vi "test Acyclic Loopback Value Overflow.vi"(8 "error in":errorcluster, 11 "TestCase in":refnum<class "Single Board Loopback.lvclass">) -> (0 "error out":errorcluster, 3 "TestCase out":refnum<class "Single Board Loopback.lvclass">)   [LabVIEW 2020, in "Single Board Loopback.lvclass"]
uses:
  Single Board Loopback.lvclass
  <vilib>/addons/_JKI Toolkits/VI Tester/TestCase.llb/TestCase.lvclass
  <vilib>/NI VeriStand/Execution/Workspace/NI_VS Workspace ExecutionAPI.lvlib
  niveristand-custom-device-testing-tools/VeriStandTestUtilities/VeriStandTestUtilities.lvlib
  <vilib>/NI VeriStand/Execution/Workspace/NI VeriStand - Set Multiple Channel Values.vi
  <vilib>/numeric/Random Number (Range) U64.vi
  C:/Users/nitest/Desktop/Git 2020/niveristand-custom-device-testing-tools/VeriStandTestCase/VeriStandTestCase.lvclass
  C:/Program Files (x86)/National Instruments/LabVIEW 2020/vi.lib/addons/_JKI Toolkits/VI Tester/TestCase.llb/TestCase.lvclass
  C:/Users/nitest/Desktop/Git 2020/niveristand-ballard-arinc429-custom-device/Source/Custom Device Support/Tests/System/Single Board Loopback/Single Board Loopback.lvclass
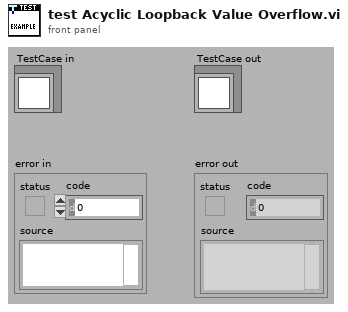
[diagram p1: front panel]
types:
  T1 = typedef "NI_VS Workspace ExecutionAPI.lvlib/WorkspaceAPI.ctl" = refnum<k24>
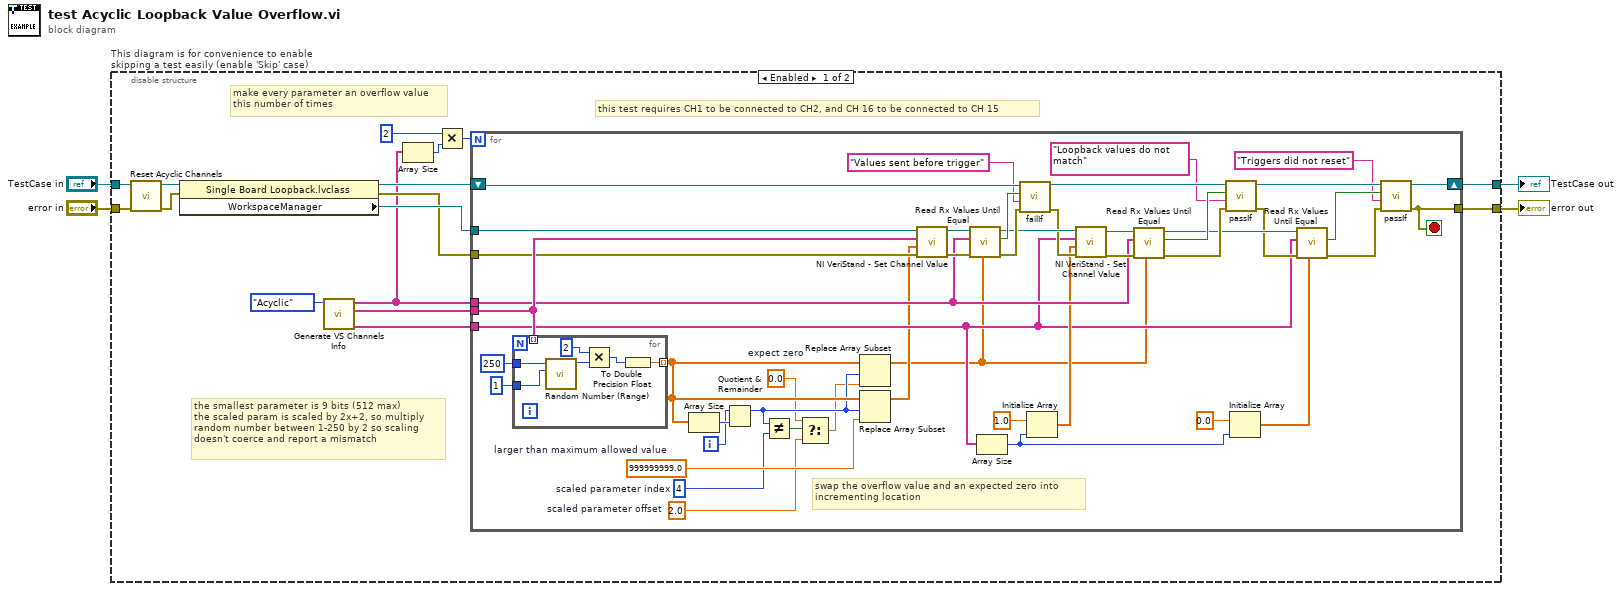
[diagram p0: block diagram]
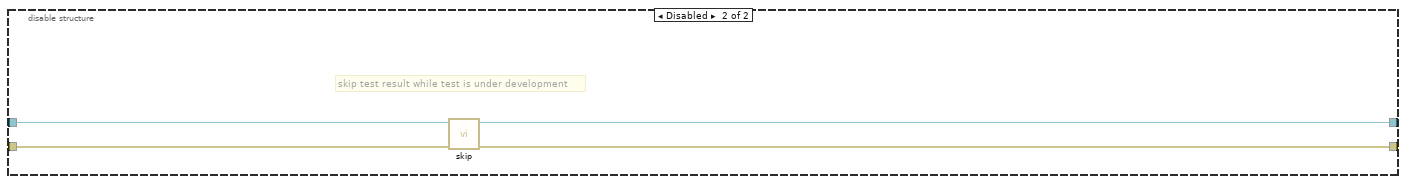
[diagram p2: hidden frame]
diagram:
  n1 = disable-structure "This diagram is for convenience to enable skipping a test easily (enable 'Skip' case)" shown="Enabled" {
    disable-tunnel: "TestCase in" -> [w5 w76]
    disable-tunnel: [w16 w74] -> w1
    disable-tunnel: [w15 w75] -> w3
    disable-tunnel: "error in" -> [w17 w73]
    frame Enabled {
      # "make every parameter an overflow value\nthis number of times"
      # "the smallest parameter is 9 bits (512 max)\nthe scaled param is scaled by 2x+2, so multiply \nrandom number between 1-250 by 2 so scaling\ndoesn't coerce and report a mismatch"
      # "this test requires CH1 to be connected to CH2, and CH 16 to be connected to CH 15"
      n2 = call "Reset Acyclic Channels.vi"("error in (no error)"=w17, "reference in"=w5) -> ("error out"=w7:errorcluster, "reference out"=w6:refnum<class "Single Board Loopback.lvclass">)  [unwired: 8 in]
      n3 = property class="Single Board Loopback.lvclass"(reference=w6, error in=w7) -> (reference out=w18:refnum<class "Single Board Loopback.lvclass">, error out=w19:errorcluster, "WorkspaceManager"=w20:T1)
      n4 = call "Generate VS Channels Info.vi"("Transfer Type"=enum16{"Acyclic", "Scheduled"}."Acyclic") -> ("Tx Trigger Channels Array"=w13:string[], "Tx Channels Array"=w14:string[], "Rx Channels Array"=w9:string[])  [unwired: 6 in, 2 out]
      n5 = Array Size(array=w9) -> (size(s)=w10:i32)
      n6 = Multiply(x=2, y=w10) -> (x*y=w12:i32)
      n7 = for {
        N: w12 -> [_]
        tunnel: w9 -> [w52]
        tunnel: w20 -> [w64]
        tunnel: w19 -> [w57]
        tunnel: w14 -> [w63]
        shift-right: [w46] -> w16
        shift-left: w18 -> [w59]
        tunnel: [w48] -> w15
        tunnel: w13 -> [w37]
        i -> [w29]
        stop <- w48 stop-if-true
        w26 = 2.0  # scaled parameter offset
        w23 = 4  # scaled parameter index
        w25 = 0.0  # expect zero
        w32 = 999999999.0  # larger than maximum allowed value
        # "swap the overflow value and an expected zero into \nincrementing location"
        n8 = for {
          tunnel: [w71] -> w30 mode=indexing
          tunnel: u64 250 ("upper bound (100)") -> [w70]
          tunnel: u64 1 ("upper bound (100)") -> [w69]
          tunnel: w63 -> [_] mode=indexing
          n9 = call-poly <vilib>:"Random Number (Range).vi"("lower bound (0)"=w69, "upper bound (100)"=w70) -> ("number"=w72:u64)  [unwired: 9 in]
          n10 = Multiply(x=u64 2, y=w72) -> (x*y=w68:u64)
          n11 = To Double Precision Float(number=w68) -> (double precision float=w71:dbl)
        }
        n12 = Array Size(array=w30) -> (size(s)=w31:i32)
        n13 = Quotient & Remainder(x=w29, y=w31) -> (x-y*floor(x/y)=w27:i32)  [unwired: 1 out]
        n14 = Not Equal?(x=w27, y=w23) -> (x != y?=w28:bool)
        n15 = Select(t=w25, s=w28, f=w26) -> (s? t:f=w24:dbl)
        n16 = Replace Array Subset(array=w30, new element=w24, index=w27) -> (w21:dbl[])
        n17 = Replace Array Subset(array=w30, new element=w32, index=w27) -> (w33:dbl[])
        n18 = call-poly <vilib>:"NI VeriStand - Set Channel Value.vi"("error in (no error)"=w57, "Values"=w33, "Channels"=w63, "WorkspaceManager in"=w64) -> ("error out"=w60:errorcluster, "WorkspaceManager out"=w62:T1)  [unwired: 6 in]
        n19 = call "Read Rx Values Until Equal.vi"("expected values"=w21, "error in"=w60, "Rx aliases"=w52, "workspace manager in"=w62) -> ("error out"=w61:errorcluster, "values equal expected"=w58:bool, "workspace manager out"=w56:T1)  [unwired: 5 in]
        n20 = Array Size(array=w37) -> (size(s)=w34:i32)
        n21 = call-dynamic "failIf.vi"("error in (no error)"=w61, "message (\"\")"="Values sent before trigger" ("message (\"\")"), "fail"=w58, "TestCase in"=w59) -> ("error out"=w55:errorcluster, "TestCase out"=w49:refnum<class "Single Board Loopback.lvclass">)  [unwired: 6 in]
        n22 = Initialize Array(1.0, w34) -> (w38:dbl[])
        n23 = call-poly <vilib>:"NI VeriStand - Set Channel Value.vi"("error in (no error)"=w55, "Values"=w38, "Channels"=w37, "WorkspaceManager in"=w56) -> ("error out"=w53:errorcluster, "WorkspaceManager out"=w54:T1)  [unwired: 6 in]
        n24 = call "Read Rx Values Until Equal.vi"("expected values"=w21, "error in"=w53, "Rx aliases"=w52, "workspace manager in"=w54) -> ("error out"=w50:errorcluster, "values equal expected"=w51:bool, "workspace manager out"=w44:T1)  [unwired: 5 in]
        n25 = call-dynamic "passIf.vi"("error in (no error)"=w50, "message (\"\")"="Loopback values do not match" ("message (\"\")"), "pass"=w51, "TestCase in"=w49) -> ("error out"=w43:errorcluster, "TestCase out"=w47:refnum<class "Single Board Loopback.lvclass">)  [unwired: 6 in]
        n26 = Initialize Array(0.0, w34) -> (w35:dbl[])
        n27 = call "Read Rx Values Until Equal.vi"("expected values"=w35, "error in"=w43, "Rx aliases"=w37, "workspace manager in"=w44) -> ("error out"=w42:errorcluster, "values equal expected"=w45:bool)  [unwired: 5 in, 1 out]
        n28 = call-dynamic "passIf.vi"("error in (no error)"=w42, "message (\"\")"="Triggers did not reset" ("message (\"\")"), "pass"=w45, "TestCase in"=w47) -> ("error out"=w48:errorcluster, "TestCase out"=w46:refnum<class "Single Board Loopback.lvclass">)  [unwired: 6 in]
      }
    }
    frame Disabled {
      # "skip test result while test is under development"
      n29 = call <vilib>:"skip.vi"("error in (no error)"=w73, "TestCase in"=w76) -> ("error out"=w75:errorcluster, "TestCase out"=w74:refnum<class "Single Board Loopback.lvclass">)  [unwired: 8 in]
    }
  }
  "error out" <- w3
  "TestCase out" <- w1
